vi "ASrreglo1disp.vi"(4 "datos":dbl[][](array[numeric]), 7 "disp. 1":i32, 10 "ARREGLO ENTRADA":dbl[][][](array[numeric])) -> (2 "output array":dbl[][][](array[numeric]))   [LabVIEW 2016]
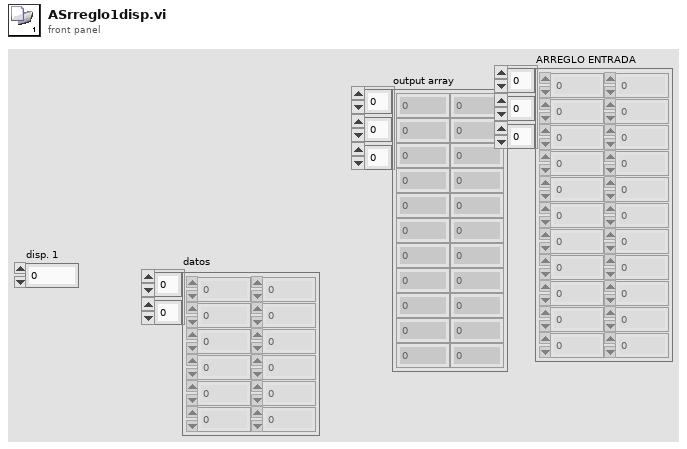
[diagram p1: front panel]
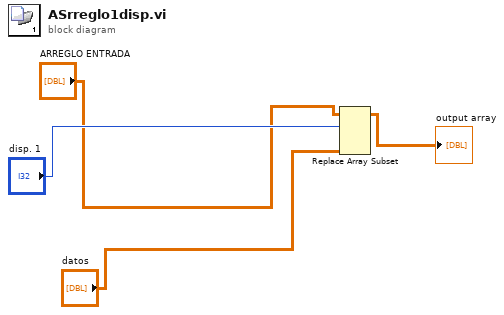
[diagram p0: block diagram]
diagram:
  n1 = Replace Array Subset(array="ARREGLO ENTRADA", new element="datos", index (dim 0)="disp. 1") -> (→"output array":dbl[][][])  [unwired: 2 in]
